vi "Init connection with server.vi"(8 "error in (no error)":errorcluster, 10 "Boolean":bool=TRUE, 11 "Control-Client in":refnum<class "Control-Client.lvclass">) -> (0 "error out":errorcluster, 3 "Control-Client out":refnum<class "Control-Client.lvclass">)   [LabVIEW 2015, in "Control-Client.lvclass"]
uses:
  Control-Client.lvclass
  Control-Client.lvclass/Control-Client.ctl
  dependecies/ControlsVIs/Clusters-def/Message types.ctl
  dependecies/ControlsVIs/Clusters-def/Commands-CLIENT.ctl
  <vilib>/NI/STM/TCP/TCP Connection Info.ctl
  <vilib>/NI/STM/SubVIs/MetaDataElement.ctl
  GeneralFunctionality/GeneralFunctionality.lvclass/GeneralFunctionality.ctl
  dependecies/ControlsVIs/Clusters-def/SERVER-Commands.ctl
  <vilib>/NI/STM/TCP/Get Connection Reference (TCP).vi
  <vilib>/NI/STM/TCP/Read Meta Data (TCP Ref).vi
  <vilib>/NI/STM/TCP/Read Meta Data (TCP Clst).vi
  Config/Config.lvclass
  dependecies/XControls/CellsDL/ControlDL.xctl
  controls/Gauge_pump/Gauge_pump.xctl
  <vilib>/NI/STM/NI STM.lvlib
  Message/Message.lvclass
  Control-Server/Control-Server.lvclass
  GeneralFunctionality/GeneralFunctionality.lvclass
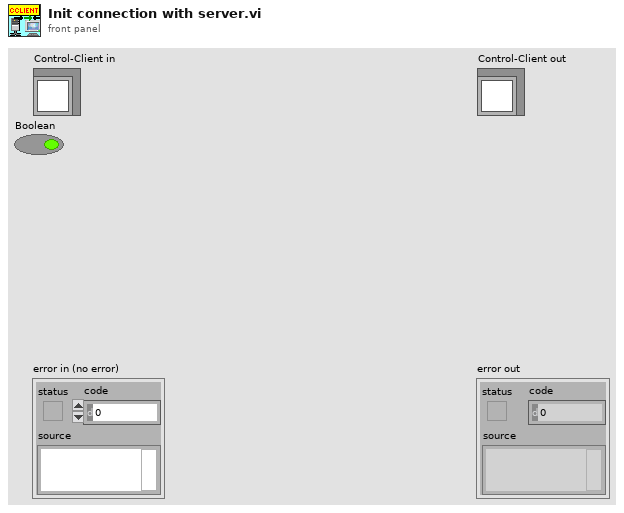
[diagram p1: front panel]
types:
  T1 = typedef "NI STM.lvlib/TCP Connection Info.ctl" = cluster{"connection ID":refnum<k5>, "meta data":T2[]}
  T2 = typedef "NI STM.lvlib/MetaDataElement.ctl" = string
  T3 = typedef "Control-Client.lvclass/Commands-CLIENT.ctl" = string
  T4 = typedef "Message types.ctl" = string
  T5 = typedef "Control-Server.lvclass/SERVER-Commands.ctl" = string
  T6 = enum8{"Enabled", "Disabled", "Disabled and Grayed Out"}
  T7 = typedef "Control-Client.lvclass/Controls-with-permissions_CLIENT.ctl" = cluster{"Server ON/OFF":refnum<vi>, "Detector connect":refnum<vi>, "DL connect":refnum<vi>, "DAQmx connect":refnum<vi>, "All connect":refnum<vi>, "Start measurement":refnum<vi>, "Move Crystal":refnum<vi>, "Relay key heater":refnum<vi>, "Laser Shutter":refnum<vi>, "Accelerator Shutter":refnum<vi>, "Power":refnum<vi>, "Unlock":refnum<vi>, "RT":refnum<vi>, "Faraday Cup":refnum<vi>, "Osc connect":refnum<vi>, "ELYSE pulses":refnum<vi>, "Cells":refnum<vi>, "ControlDL":refnum<vi>, "Pump":refnum<vi>, "# par point":refnum<vi>, "Alarm":refnum<vi>, "oscilloscopeRead":refnum<vi>, "WCM_state":refnum<vi>}
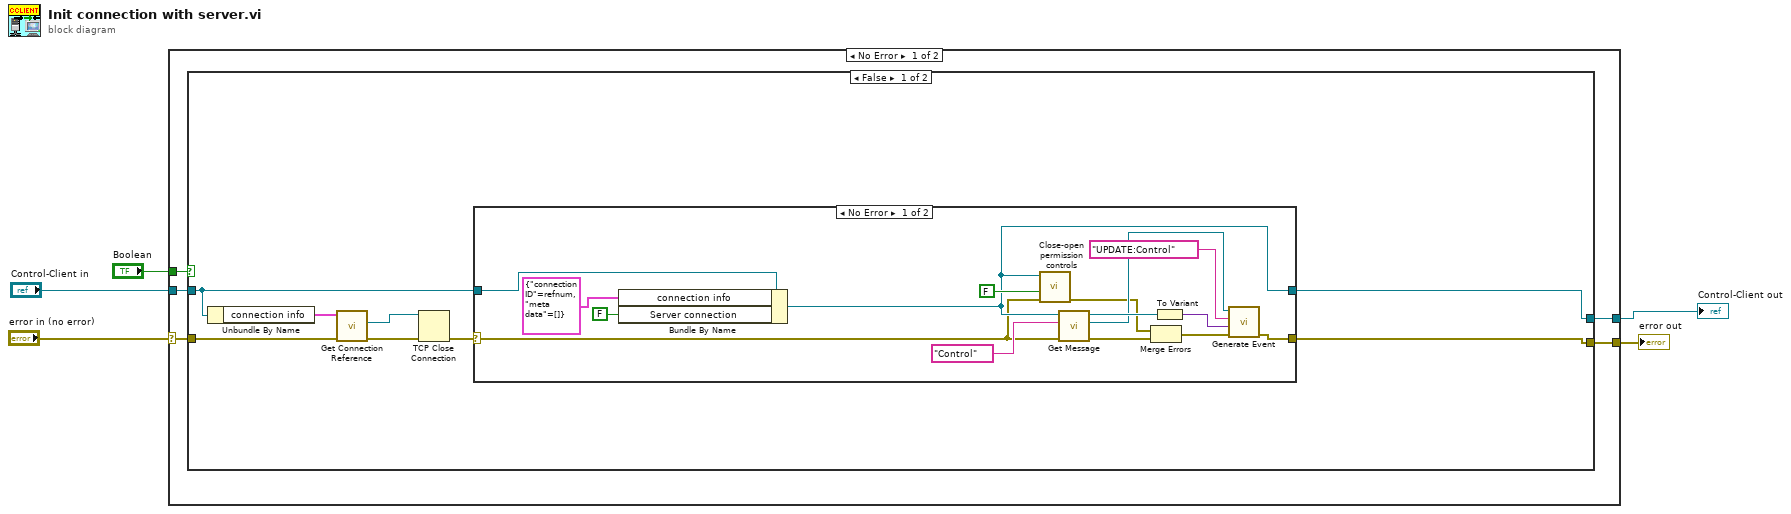
[diagram p0: block diagram]
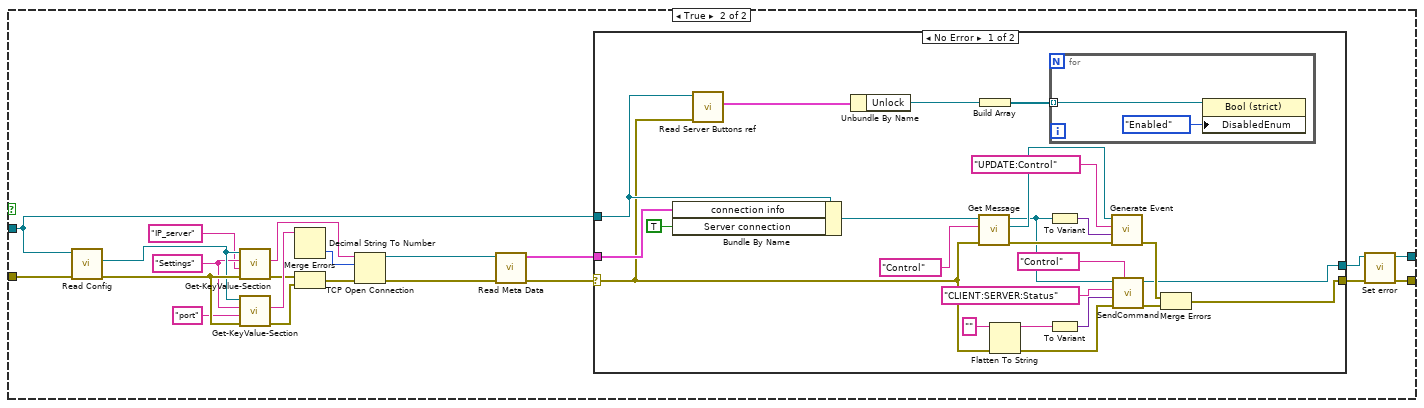
[diagram p3: hidden frame]
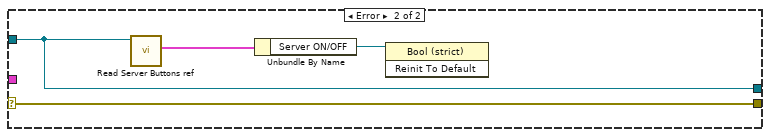
[diagram p4: hidden frame]
diagram:
  n1 = case shown="No Error" "error in (no error)" {
    selector: "error in (no error)" -> [w10 w88]
    tunnel: [w7 w88] -> w4
    tunnel: [w8 w87] -> w2
    tunnel: "Control-Client in" -> [w9 w87]
    tunnel: "Boolean" -> [w6 _]
    frame No Error {
      n2 = case shown="False" w6 {
        tunnel: w10 -> [w16 w54]
        tunnel: w9 -> [w14 w41]
        tunnel: [w13 w38] -> w8
        tunnel: [w11 w36] -> w7
        frame False {
          n3 = Unbundle By Name(w14) -> ("connection info"=w18:T1)
          n4 = call-poly <vilib>:"Get Connection Reference.vi"("error in"=w16, "connection info in"=w18) -> ("error out"=w15:errorcluster, "connection ID out"=w17:refnum<k5>)  [unwired: 7 in, 1 out]
          n5 = TCP Close Connection(connection ID=w17, error in (no error)=w15) -> (error out=w12:errorcluster)  [unwired: 1 in, 1 out]
          n6 = case shown="No Error" w12 {
            selector: w12 -> [w20 w35]
            tunnel: [w21 w34] -> w13
            tunnel: [w19 w35] -> w11
            tunnel: w14 -> [w26 w34]
            frame No Error {
              n7 = Bundle By Name(cluster=w26, "connection info"=T1 {"connection ID"=refnum, "meta data"=[]}, "Server connection"=FALSE) -> (w21:refnum<class "Control-Client.lvclass">)
              n8 = call "Close-open permission controls.vi"("error in (no error)"=w20, "Boolean"=FALSE, "Control-Client in"=w21) -> ("error out"=w25:errorcluster)  [unwired: 7 in, 1 out]
              n9 = call "Get Message.vi"("error in (no error)"=w20, "Message type"=T4 "Control", "GeneralFunctionality en entrée"=w21) -> ("error out"=w24:errorcluster, "Message.lvclass"=w30:refnum<class "Message.lvclass">, "GeneralFunctionality en sortie"=w32:refnum<class "Control-Client.lvclass">)  [unwired: 6 in]
              n10 = Merge Errors(w25, w24) -> (w23:errorcluster)
              n11 = To Variant(anything=w32) -> (Variant=w28:variant)
              n12 = call "Generate Event.vi"("error in (no error)"=w23, "Data"=w28, "Command"=T3 "UPDATE:Control" ("Commands-Client"), "Message en entrée"=w30) -> ("error out"=w19:errorcluster)  [unwired: 6 in, 1 out]
            }
            frame Error {
            }
          }
        }
        frame True {
          w51 = "Settings" ("Section")
          n13 = call "Read Config.vi"("error in (no error)"=w54, "GeneralFunctionality en entrée"=w41) -> ("error out"=w53:errorcluster, "Config.lvclass"=w52:refnum<class "Config.lvclass">)  [unwired: 7 in, 1 out]
          n14 = call-dynamic "Get-KeyValue-Section.vi"("error in (no error)"=w53, "Key"="IP_server", "Section"=w51, "Config in"=w52) -> ("error out"=w45:errorcluster, "Value"=w49:string)  [unwired: 5 in, 1 out]
          n15 = call-dynamic "Get-KeyValue-Section.vi"("error in (no error)"=w53, "Key"="port", "Section"=w51, "Config in"=w52) -> ("error out"=w44:errorcluster, "Value"=w47:string)  [unwired: 5 in, 1 out]
          n16 = Decimal String To Number(string=w47) -> (number=w46:i32)  [unwired: 2 in, 1 out]
          n17 = Merge Errors(w45, w44) -> (w43:errorcluster)
          n18 = TCP Open Connection(address=w49, remote port or service name=w46, error in (no error)=w43) -> (connection ID=w56:refnum<k5>, error out=w55:errorcluster)  [unwired: 2 in]
          n19 = call-poly <vilib>:"Read Meta Data.vi"("error in"=w55, "connection ID"=w56) -> ("error out"=w42:errorcluster, "connection info out"=w40:T1)  [unwired: 7 in, 1 out]
          n20 = case shown="No Error" w42 {
            selector: w42 -> [w66 w86]
            tunnel: w41 -> [w74 w85]
            tunnel: [w57 w85] -> w39
            tunnel: w40 -> [w80 _]
            tunnel: [w70 w86] -> w37
            frame No Error {
              n21 = Bundle By Name(cluster=w74, "connection info"=w80, "Server connection"=TRUE) -> (w59:refnum<class "Control-Client.lvclass">)
              n22 = call "Read Server Buttons ref.vi"("error in (no error)"=w66, "Control-Client in"=w74) -> ("Server Buttons ref"=w75:T7)  [unwired: 7 in, 2 out]
              n23 = Unbundle By Name(w75) -> ("Unlock"=w73:refnum<vi>)
              n24 = call "Get Message.vi"("error in (no error)"=w66, "Message type"=T4 "Control", "GeneralFunctionality en entrée"=w59) -> ("error out"=w68:errorcluster, "Message.lvclass"=w69:refnum<class "Message.lvclass">, "GeneralFunctionality en sortie"=w58:refnum<class "Control-Client.lvclass">)  [unwired: 6 in]
              n25 = Build Array(w73) -> (w72:refnum<vi>[])
              n26 = Flatten To String(anything="", error in (no error)=w66) -> (data string=w61:string, error out=w62:errorcluster)  [unwired: 2 in, 1 out]
              n27 = for {
                tunnel: w72 -> [w81] mode=indexing
                n28 = property class="Bool (strict)"(reference=w81, "DisabledEnum"=T6."Enabled" ("Désactivé")) -> ()  [unwired: 1 in, 2 out]
              }
              n29 = To Variant(anything=w58) -> (Variant=w76:variant)
              n30 = To Variant(anything=w61) -> (Variant=w64:variant)
              n31 = call "Generate Event.vi"("error in (no error)"=w68, "Data"=w76, "Command"=T3 "UPDATE:Control" ("Commands-Client"), "Message en entrée"=w69) -> ("error out"=w71:errorcluster)  [unwired: 6 in, 1 out]
              n32 = call "SendCommand.vi"("Message type"=T4 "Control", "error in (no error)"=w62, "data"=w64, "Command"=T5 "CLIENT:SERVER:Status" ("Commands"), "Control-Client in"=w58) -> ("error out"=w65:errorcluster, "Control-Client out"=w57:refnum<class "Control-Client.lvclass">)  [unwired: 5 in]
              n33 = Merge Errors(w71, w65) -> (w70:errorcluster)
            }
            frame Error {
              n34 = call "Read Server Buttons ref.vi"("Control-Client in"=w85) -> ("Server Buttons ref"=w84:T7)  [unwired: 8 in, 2 out]
              n35 = Unbundle By Name(w84) -> ("Server ON/OFF"=w83:refnum<vi>)
              n36 = invoke class="Bool (strict)" method="Reinit To Default"(reference=w83) -> ()  [unwired: 2 in, 3 out]
            }
          }
          n37 = call "Set error.vi"("error in (no error)"=w37, "Control-Client in"=w39) -> ("error out"=w36:errorcluster, "Control-Client out"=w38:refnum<class "Control-Client.lvclass">)  [unwired: 8 in]
        }
      }
    }
    frame Error {
    }
  }
  "error out" <- w4
  "Control-Client out" <- w2
